vi "get_1000m_flags.vi"(3 "flag-timestamp array":cluster{"String":string, timestamp}[](array[cluster])) -> (0 "1000 m start":timestamp, 1 "1000 m end":timestamp)   [LabVIEW 2020]
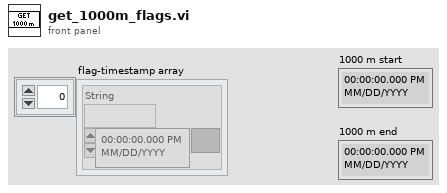
[diagram p1: front panel]
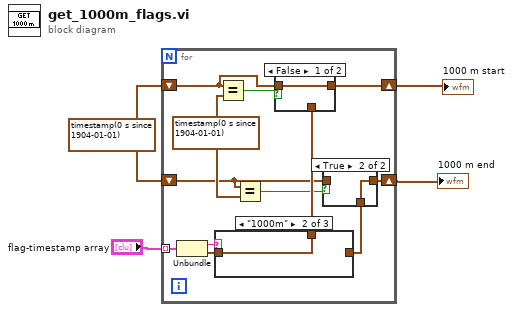
[diagram p0: block diagram]
diagram:
  w3 = timestamp(0 s since 1904-01-01)
  n1 = for {
    shift-right: [w11] -> w4
    shift-left: w3 -> [w10]
    shift-right: [w8] -> w1
    shift-left: w3 -> [w5]
    tunnel: "flag-timestamp array" -> [w16] mode=indexing
    w6 = timestamp(0 s since 1904-01-01)
    n2 = Unbundle(w16) -> ("String"=w15:string, w14:timestamp)
    n3 = case shown="\"1000m\"" w15 {
      tunnel: w14 -> [_ w21 w22]
      tunnel: [_ w21 _] -> w12
      tunnel: [_ _ w22] -> w9
      frame Default {
      }
      frame "1000m" {
      }
      frame "1000m_end" {
      }
    }
    n4 = Equal?(x=w10, y=w6) -> (x = y?=w13:bool)
    n5 = Equal?(x=w5, y=w6) -> (x = y?=w7:bool)
    n6 = case shown="False" w13 {
      tunnel: w12 -> [_ w20]
      tunnel: [w19 w20] -> w11
      tunnel: w10 -> [w19 _]
      frame False {
      }
      frame True {
      }
    }
    n7 = case shown="True" w7 {
      tunnel: w9 -> [_ w18]
      tunnel: [w17 w18] -> w8
      tunnel: w5 -> [w17 _]
      frame False {
      }
      frame True {
      }
    }
  }
  "1000 m start" <- w4
  "1000 m end" <- w1
